vi "IndexControl.vi"(8 "Power":dbl, 10 "Backward":bool, 11 "Forward":bool) -> (2 "Numeric":dbl)   [LabVIEW 2011]
uses:
  System Set Points and States.vi
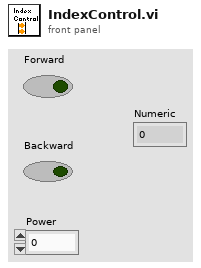
[diagram p1: front panel]
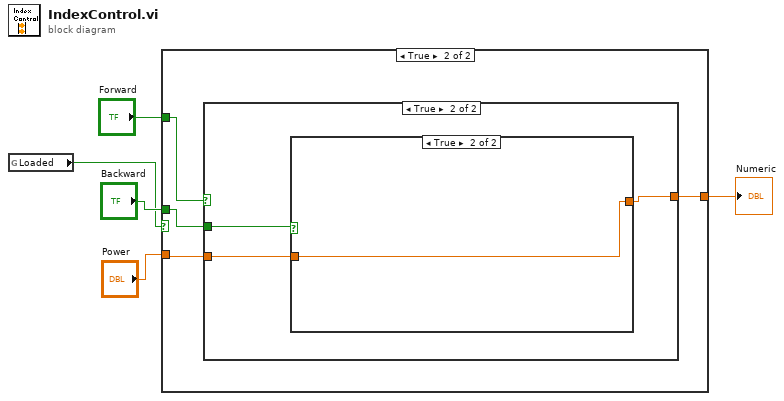
[diagram p0: block diagram]
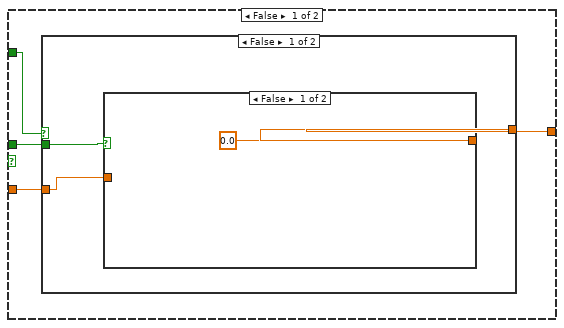
[diagram p2: hidden frame]
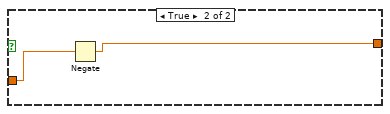
[diagram p3: hidden frame]
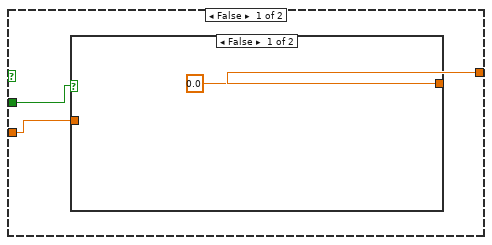
[diagram p5: hidden frame]
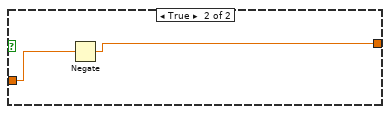
[diagram p6: hidden frame]
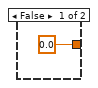
[diagram p7: hidden frame]
diagram:
  n1 = global read "System Set Points and States.vi" "Loaded"() -> (w1:bool)
  n2 = case shown="True" w1 {
    tunnel: "Forward" -> [w9 w18]
    tunnel: "Power" -> [w8 w19]
    tunnel: [w7 w20] -> w3
    tunnel: "Backward" -> [w6 w17]
    frame False {
      n3 = case shown="False" w9 {
        tunnel: w8 -> [w11 w16]
        tunnel: [w10 w16] -> w7
        tunnel: w6 -> [w12 _]
        frame False {
          n4 = case shown="False" w12 {
            tunnel: w11 -> [_ w15]
            tunnel: [0.0 w14] -> w10
            frame False {
            }
            frame True {
              n5 = Negate(x=w15) -> (-x=w14:dbl)
            }
          }
        }
        frame True {
        }
      }
    }
    frame True {
      n6 = case shown="True" w18 {
        tunnel: w19 -> [w23 w27]
        tunnel: [w22 w29] -> w20
        tunnel: w17 -> [w21 w28]
        frame False {
          n7 = case shown="False" w21 {
            tunnel: w23 -> [_ w26]
            tunnel: [0.0 w25] -> w22
            frame False {
            }
            frame True {
              n8 = Negate(x=w26) -> (-x=w25:dbl)
            }
          }
        }
        frame True {
          n9 = case shown="True" w28 {
            tunnel: [0.0 w31] -> w29
            tunnel: w27 -> [_ w31]
            frame False {
            }
            frame True {
            }
          }
        }
      }
    }
  }
  "Numeric" <- w3
